vi "Create Score File.vi"(8 "Submitter":string, 9 "GUID":u16, 10 "Round":u16, 11 "Scoring Data":cluster{"Name":string, "Value":string}[](array[cluster])) -> ()   [LabVIEW 2013]
uses:
  Score File Queue Contents.ctl
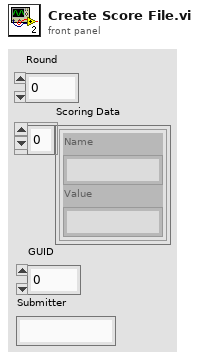
[diagram p1: front panel]
types:
  T1 = typedef "Score File Queue Contents.ctl" = cluster{"Scoring Data":cluster{"Name":string, "Value":string}[], "Round":u16, "GUID":u16, "GUSID":string, "Time Stamp":timestamp, "Submitter":string}
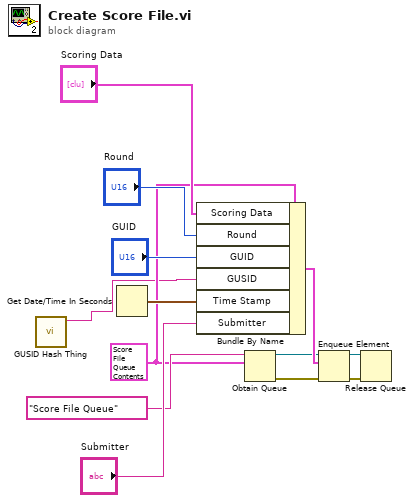
[diagram p0: block diagram]
diagram:
  w7 = T1 {"Scoring Data"=[], "Round"=0, "GUID"=0, "GUSID"="", "Time Stamp"=timestamp(0 s since 1904-01-01), "Submitter"=""} ("Cluster")
  n1 = call "GUSID Hash Thing.vi"() -> ("String"=w1:string)  [unwired: 11 in]
  n2 = Get Date/Time In Seconds() -> (seconds since 1Jan1904=w13:timestamp)
  n3 = Bundle By Name(cluster=w7, "Scoring Data"="Scoring Data", "Round"="Round", "GUID"="GUID", "GUSID"=w1, "Time Stamp"=w13, "Submitter"="Submitter") -> (w5:T1)
  n4 = Obtain Queue(name (unnamed)="Score File Queue", element data type=w7) -> (queue out=w4:refnum<queue>, error out=w6:errorcluster)  [unwired: 3 in, 1 out]
  n5 = Enqueue Element(queue=w4, element=w5, error in (no error)=w6) -> (queue out=w3:refnum<queue>, error out=w2:errorcluster)  [unwired: 1 in, 1 out]
  n6 = Release Queue(queue=w3, error in (no error)=w2) -> ()  [unwired: 1 in, 3 out]
